vi "Panel Delete From Subpanel.vi"(8 "error in (no error)":errorcluster, 11 "Panel Control_Ref in":refnum<class "Panel Controller.lvclass">) -> (0 "error out":errorcluster, 3 "Panel Control_Ref out":refnum<class "Panel Controller.lvclass">)   [LabVIEW 2015, in "Panel Controller.lvclass"]
uses:
  Panel Controller.lvclass
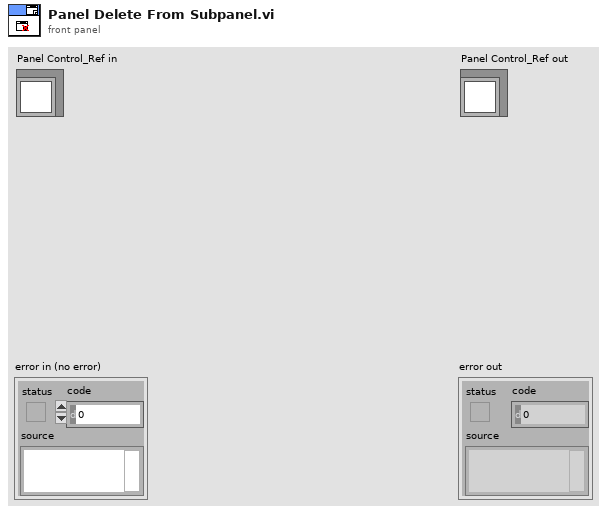
[diagram p1: front panel]
types:
  T1 = typedef "Panel Controller.lvclass/ObjectAttributes.ctl" = cluster{"Sub Panel Ref":refnum<vi>, "Panel_Q":refnum<queue>, "VI Running Refnum":refnum<vi>, "Brower Controller_Q":refnum<class "Message Enqueuer.lvclass">, "GUI Control Builder Director.lvclass":refnum<class "GUI Control Builder Director.lvclass">, "Panel GUI Manager.lvclass":refnum<class "Panel GUI Manager.lvclass">}
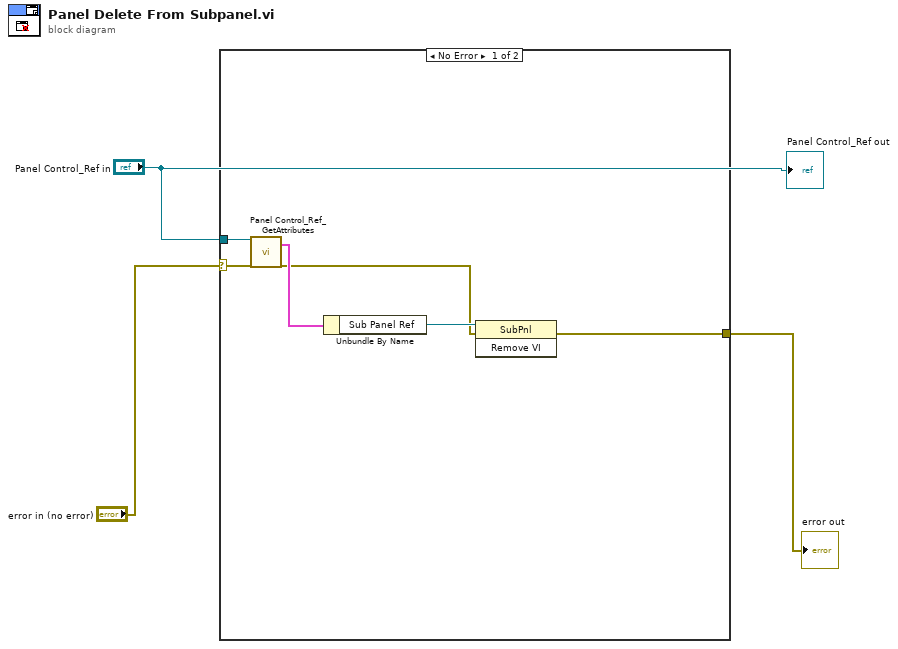
[diagram p0: block diagram]
diagram:
  n1 = case shown="No Error" "error in (no error)" {
    selector: "error in (no error)" -> [w9 w10]
    tunnel: [w5 w10] -> w2
    tunnel: "Panel Control_Ref in" -> [w4 _]
    frame No Error {
      n2 = call "Panel Control_Ref_GetAttributes.vi"("reference in"=w4, "error in (no error)"=w9) -> ("Data"=w8:T1, "error out"=w6:errorcluster)  [unwired: 14 in, 2 out]
      n3 = Unbundle By Name(w8) -> ("Sub Panel Ref"=w7:refnum<vi>)
      n4 = invoke class="SubPnl" method="Remove VI"(reference=w7, error in=w6) -> (error out=w5:errorcluster)  [unwired: 1 in, 2 out]
    }
    frame Error {
    }
  }
  "error out" <- w2
  "Panel Control_Ref out" <- "Panel Control_Ref in"
